vi "Latch and Hold.vi"(10 "Clear":bool, 11 "Valid":bool) -> (3 "Output":bool)   [LabVIEW 2015]
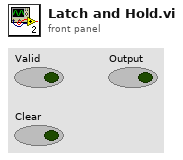
[diagram p1: front panel]
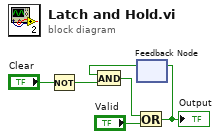
[diagram p0: block diagram]
diagram:
  n1 = Not(x="Clear") -> (.not. x?=w1:bool)
  n2 = feedback #1() -> (w5:bool)  [unwired: 1 in]
  n3 = And(x=w5, y=w1) -> (x .and. y?=w6:bool)
  n4 = Or(x=w6, y="Valid") -> (x .or. y?=w4:bool)
  "Output" <- w4
  n5 = feedback-in #1(w4) -> ()
